vi "Symphony Read Det Uniq_ID.vi"(8 "error in (no error)":errorcluster) -> (0 "error out":errorcluster, 1 "Name":string[](array[string]), 2 "DeviceName":string[](array[string]), 3 "UniqueID":string[](array[string]), 4 "nbr of components":i32)   [LabVIEW 2019]
uses:
  <vilib>/registry/registry.llb/Registry RtKey.ctl
  <vilib>/registry/registry.llb/Read Registry Value Simple STR.vi
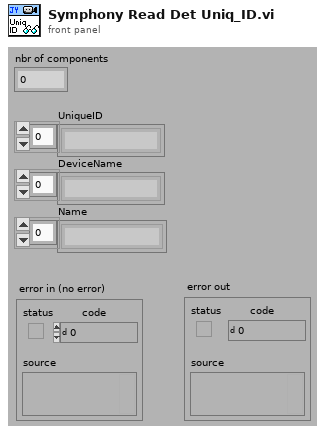
[diagram p1: front panel]
types:
  T1 = enum16{"ReadRegKeys", "GetCCDKeys", "ReadKeyData", "Error"}
  T2 = typedef "Registry RtKey.ctl" = enum32{"HKEY_CLASSES_ROOT", "HKEY_CURRENT_USER", "HKEY_LOCAL_MACHINE", "HKEY_USERS", "HKEY_PERFORMANCE_DATA", "HKEY_CURRENT_CONFIG", "HKEY_DYN_DATA"}
  T3 = typedef "Registry refnum.ctl" = refnum<k1>
  T4 = cluster{"numSubKeys":i32, "maxSubKeyLen":i32, "maxSubKeyClassLen":i32}
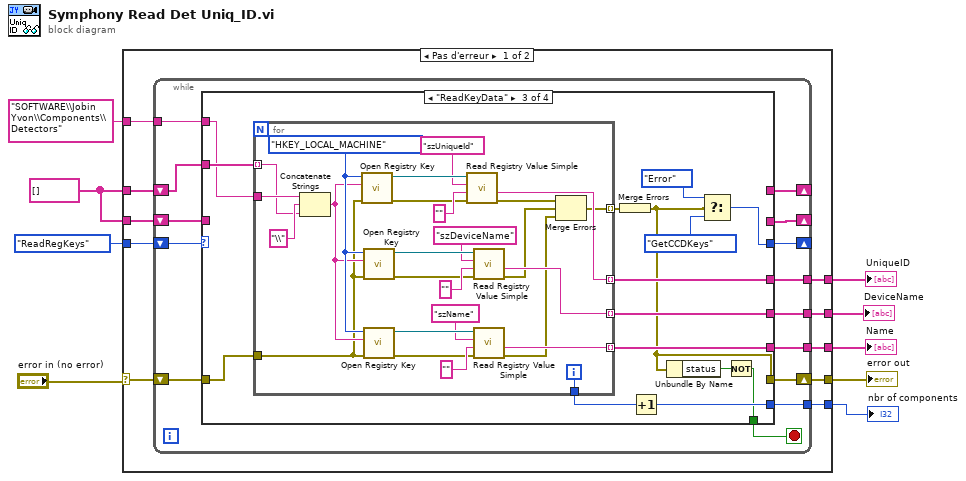
[diagram p0: block diagram]
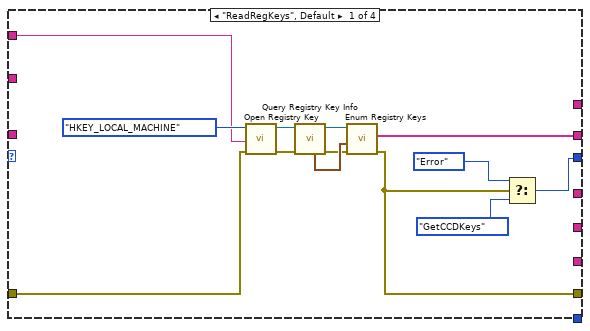
[diagram p2: hidden frame]
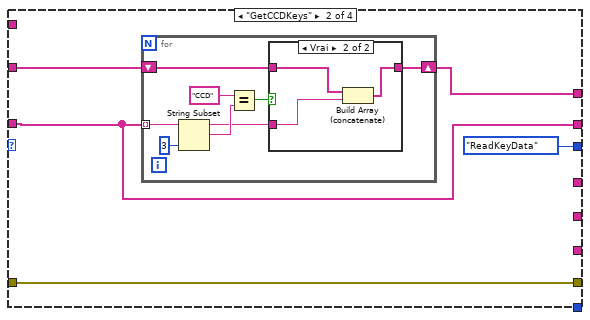
[diagram p3: hidden frame]
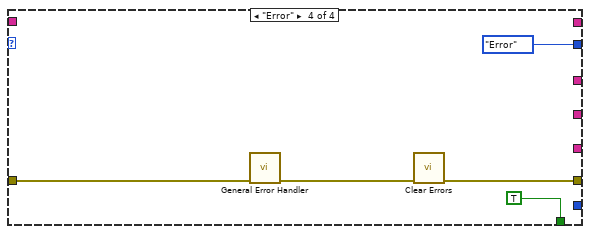
[diagram p5: hidden frame]
diagram:
  w7 = string[] [] ("test")
  n1 = case shown="Pas d'erreur" "error in (no error)" {
    selector: "error in (no error)" -> [w17 w109]
    tunnel: T1."ReadRegKeys" -> [w19 _]
    tunnel: w7 -> [w18 _]
    tunnel: w7 -> [w16 _]
    tunnel: [w15 _] -> w6
    tunnel: [w14 w109] -> w5
    tunnel: [w13 _] -> w4
    tunnel: [w12 _] -> w3
    tunnel: [w11 _] -> w2
    tunnel: "SOFTWARE\\Jobin Yvon\\Components\\Detectors" ("subkey") -> [w10 _]
    frame No Error {
      n2 = while {
        shift-right: [w25] -> _
        shift-left: w19 -> [w32]
        shift-right: [w28] -> _
        shift-left: w18 -> [w31]
        shift-right: [w27] -> w14
        shift-left: w17 -> [w33]
        shift-right: [w30] -> _
        shift-left: w16 -> [w29]
        tunnel: [w26] -> w15
        tunnel: [w24] -> w13
        tunnel: [w23] -> w12
        tunnel: [w22] -> w11
        tunnel: w10 -> [w20]
        stop <- w21 stop-if-true
        n3 = case shown="\"ReadKeyData\"" w32 {
          tunnel: w33 -> [w39 w47 w77 w107]
          tunnel: w31 -> [_ w51 w74 _]
          tunnel: [w40 w49 _ _] -> w30
          tunnel: w29 -> [_ w49 _ _]
          tunnel: [_ w50 _ _] -> w28
          tunnel: [w38 w47 w66 w105] -> w27
          tunnel: [_ _ w75 _] -> w26
          tunnel: [w35 T1."ReadKeyData" w69 T1."Error"] -> w25
          tunnel: [_ _ w72 _] -> w24
          tunnel: [_ _ w68 _] -> w23
          tunnel: [_ _ w67 _] -> w22
          tunnel: [_ _ w64 TRUE] -> w21
          tunnel: w20 -> [w34 _ w63 _]
          frame "ReadRegKeys", Default {
            n4 = call <vilib>:"Open Registry Key.vi"("error in (no error)"=w39, "subkey"=w34, "root key (HKEY_LOCAL_MACHINE)"=Registry_RtKey."HKEY_LOCAL_MACHINE") -> ("error out"=w44:errorcluster, "refnum out"=w45:T3)  [unwired: 7 in]
            n5 = call <vilib>:"Query Registry Key Info.vi"("error in (no error)"=w44, "refnum"=w45) -> ("error out"=w42:errorcluster, "refnum out"=w41:T3, "subkey info"=w46:T4)  [unwired: 5 in, 2 out]
            n6 = call <vilib>:"Enum Registry Keys.vi"("error in (no error)"=w42, "subkey info"=w46, "refnum"=w41) -> ("error out"=w38:errorcluster, "subkeys"=w40:string[])  [unwired: 6 in, 1 out]
            n7 = Select(t=T1."Error", s=w38, f=T1."GetCCDKeys") -> (s? t:f=w35:T1)
          }
          frame "GetCCDKeys" {
            n8 = for {
              tunnel: w49 -> [w54] mode=indexing
              shift-right: [w52] -> w50
              shift-left: w51 -> [w53]
              n9 = String Subset(string=w54, length (rest)=3 ("longueur (reste)")) -> (substring=w55:string)  [unwired: 1 in]
              n10 = Equal?(x="CCD", y=w55) -> (x = y?=w56:bool)
              n11 = case shown="Vrai" w56 {
                tunnel: w54 -> [_ w62]
                tunnel: w53 -> [w59 w61]
                tunnel: [w59 w60] -> w52
                frame False {
                }
                frame True {
                  n12 = Build Array (concatenate)(w61, w62) -> (w60:string[])
                }
              }
            }
          }
          frame "ReadKeyData" {
            n13 = for {
              tunnel: w74 -> [w83] mode=indexing
              tunnel: w63 -> [w101]
              tunnel: [w102] -> w75 mode=indexing
              tunnel: [w88] -> w68 mode=indexing
              tunnel: [w87] -> w67 mode=indexing
              tunnel: [w86] -> w73
              tunnel: w77 -> [w82]
              tunnel: [w78] -> w76 mode=indexing
              i -> [w86]
              w89 = Registry_RtKey."HKEY_LOCAL_MACHINE" ("root key (HKEY_LOCAL_MACHINE)")
              n14 = Concatenate Strings(w101, "\\" ("Sous-chaîne"), w83) -> (w85:string)
              n15 = call <vilib>:"Open Registry Key.vi"("error in (no error)"=w82, "subkey"=w85, "root key (HKEY_LOCAL_MACHINE)"=w89) -> ("error out"=w99:errorcluster, "refnum out"=w100:T3)  [unwired: 7 in]
              n16 = call <vilib>:"Open Registry Key.vi"("error in (no error)"=w82, "subkey"=w85, "root key (HKEY_LOCAL_MACHINE)"=w89) -> ("error out"=w95:errorcluster, "refnum out"=w96:T3)  [unwired: 7 in]
              n17 = call <vilib>:"Open Registry Key.vi"("error in (no error)"=w82, "subkey"=w85, "root key (HKEY_LOCAL_MACHINE)"=w89) -> ("error out"=w91:errorcluster, "refnum out"=w92:T3)  [unwired: 7 in]
              n18 = call-poly <vilib>:"Read Registry Value Simple.vi"("error in (no error)"=w99, "default data"="", "value"="szUniqueId" ("Sous-chaîne"), "refnum"=w100) -> ("error out"=w81:errorcluster, "String/Binary data"=w102:string)  [unwired: 2 in, 2 out]
              n19 = call-poly <vilib>:"Read Registry Value Simple.vi"("error in (no error)"=w95, "default data"="", "value"="szDeviceName", "refnum"=w96) -> ("error out"=w80:errorcluster, "String/Binary data"=w88:string)  [unwired: 2 in, 2 out]
              n20 = call-poly <vilib>:"Read Registry Value Simple.vi"("error in (no error)"=w91, "default data"="", "value"="szName", "refnum"=w92) -> ("error out"=w79:errorcluster, "String/Binary data"=w87:string)  [unwired: 2 in, 2 out]
              n21 = Merge Errors(w81, w80, w79) -> (w78:errorcluster)
            }
            n22 = Merge Errors(w76) -> (w66:errorcluster)
            n23 = Increment(x=w73) -> (x+1=w72:i32)
            n24 = Unbundle By Name(w66) -> ("status"=w65:bool)
            n25 = Select(t=T1."Error", s=w66, f=T1."GetCCDKeys") -> (s? t:f=w69:T1)
            n26 = Not(x=w65) -> (.not. x?=w64:bool)
          }
          frame "Error" {
            n27 = call <vilib>:"General Error Handler.vi"("error in (no error)"=w107) -> ("error out"=w106:errorcluster)  [unwired: 10 in, 4 out]
            n28 = call <vilib>:"Clear Errors.vi"("error in (no error)"=w106) -> ("error out"=w105:errorcluster)  [unwired: 5 in, 1 out]
          }
        }
      }
    }
    frame Error {
    }
  }
  "error out" <- w5
  "Name" <- w2
  "DeviceName" <- w3
  "UniqueID" <- w6
  "nbr of components" <- w4
